vi "MQTT Basics -- Low Level.vi"() -> ()   [LabVIEW 2019]
uses:
  <vilib>/LabVIEW Open Source Project/MQTT Control Packets/Control Packets/CONNECT/Create CONNECT Packet.vi
  <vilib>/LabVIEW Open Source Project/MQTT Control Packets/Control Packets/CONNECT/CONNECT.lvclass
  <vilib>/LabVIEW Open Source Project/MQTT Control Packets/Control Packets/ControlPacket/ControlPacket.lvclass
  <vilib>/LabVIEW Open Source Project/MQTT Control Packets/Control Packets/MQTT_311/MQTTVersion.lvclass
  <vilib>/LabVIEW Open Source Project/MQTT Control Packets/Control Packets/CONNACK/CONNACK.lvclass
  <vilib>/LabVIEW Open Source Project/MQTT Control Packets/Control Packets/CONNACK/Connect Return Code -- enum.ctl
panel:
  out "Return Code":T1=enum."Server Unavailable"
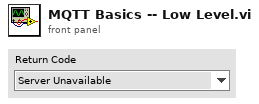
[diagram p1: front panel]
types:
  T1 = typedef "MQTT_Control_Packets.lvlib/CONNACK.lvclass/Connect Return Code -- enum.ctl" = enum16{"Connection accepted", "Unacceptable protocol version", "Identifier Rejected", "Server Unavailable", "Bad Username or Password", "Not Authorized"}
  T2 = enum16{"Standard", "Buffered", "CRLF", "Immediate"}
  T3 = typedef "MQTT_Control_Packets.lvlib/ControlPacket.lvclass/Control Packet Type -- enum.ctl" = enum16{"Reserved", "CONNECT", "CONNACK", "PUBLISH", "PUBACK", "PUBREC", "PUBREL", "PUBCOMP", "SUBSCRIBE", "SUBACK", "UNSUBSCRIBE", "UNSUBACK", "PINGREQ", "PINGRESP", "DISCONNECT", "AUTH"}
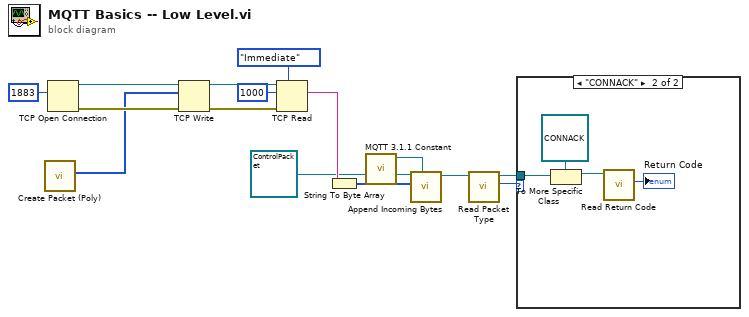
[diagram p0: block diagram]
diagram:
  n1 = call-poly <vilib>:"Create Packet (Poly).vi"() -> ("Bytes Stream"=w1:u8[])  [unwired: 9 in, 2 out]
  n2 = TCP Open Connection(remote port or service name=u16 1883) -> (connection ID=w6:refnum<k5>, error out=w5:errorcluster)  [unwired: 4 in]
  n3 = TCP Write(connection ID=w6, data in=w1, error in (no error)=w5) -> (connection ID out=w15:refnum<k5>, error out=w4:errorcluster)  [unwired: 1 in, 1 out]
  n4 = TCP Read(connection ID=w15, bytes to read=1000, error in (no error)=w4, 7:T2."Immediate" ("mode (standard)")) -> (data out=w14:string)  [unwired: 1 in, 2 out]
  n5 = String To Byte Array(string=w14) -> (unsigned byte array=w12:u8[])
  n6 = call <vilib>:"MQTT 3.1.1 Constant.vi"() -> ("MQTT 3.1.1"=w13:refnum<class "MQTTVersion.lvclass">)  [unwired: 11 in]
  n7 = call <vilib>:"Append Incoming Bytes.vi"("MQTT Version (3.1.1)"=w13, "Incoming Packets"=w12, "Incomplete ControlPacket"=refnum<class "ControlPacket.lvclass"> refnum) -> ("ControlPacket"=w11:refnum<class "ControlPacket.lvclass">)  [unwired: 5 in, 3 out]
  n8 = call <vilib>:"Read Packet Type.vi"("ControlPacket in"=w11) -> ("Control Packet Type"=w10:T3, "ControlPacket out"=w9:refnum<class "ControlPacket.lvclass">)  [unwired: 9 in]
  n9 = case shown="\"CONNACK\"" w10 {
    tunnel: w9 -> [_ w19]
    frame "Reserved", Default {
    }
    frame "CONNACK" {
      n10 = To More Specific Class(target class=refnum<class "CONNACK.lvclass"> refnum ("CONNACK in"), reference=w19) -> (specific class reference=w17:refnum<class "CONNACK.lvclass">)  [unwired: 1 in, 1 out]
      n11 = call <vilib>:"Read Return Code.vi"("CONNACK in"=w17) -> ("Return Code"=→"Return Code":T1)  [unwired: 8 in, 2 out]
    }
  }
